vi "Fetch Multi Eval Meas List SEM Margin Area Results.vi"(6 "Area (1)":T2=1, 7 "Offset Frequency (Negative)":i32(ring) items=["Negative", "Positive"], 8 "error in (no error)":errorcluster, 9 "Result Type (Current)":i32(ring) items=["Current"=0, "Average"=1, "Minimum"=5], 10 "Instance (1)":T3=1, 11 "VISA resource name":refnum<visa-resource-name>) -> (0 "error out":errorcluster, 2 "Reliability":i32, 3 "VISA resource name out":refnum<visa-resource-name>)   [LabVIEW 2020, in "Rohde&Schwarz CMXP NR FR2 Measurement.lvlib"]
doc: "Returns spectrum emission mask margin positions for all measured list mode segments.\n\nAttributes:\nRSCMXPNRFR2M_ATTR_FETCH_MULTI_EVAL_MEASUREMENT_LIST_SEM_MARGIN_AREA_NEGATIVE_AVERAGE_RESULTS\nRSCMXPNRFR2M_ATTR_FETCH_MULTI_EVAL_MEASUREMENT_LIST_SEM_MARGIN_AREA_NEGATIVE_CURRENT_RESULTS\nRSCMXPNRFR2M_ATTR_FETCH_MULTI_EVAL_MEASUREMENT_LIST_SEM_MARGIN_AREA_NEGATIVE_MINIMUM_RESULTS\nRSCMXPNRFR2M_ATTR_FETCH_MULTI_EVAL_MEASUREMENT_LIST_SEM_MARGIN_AREA_POSITIVE_AVERAGE_RESULTS\nRSCMXPNRFR2M_ATTR_FETCH_MULTI_EVAL_MEASUREMENT_LIST_SEM_MARGIN_AREA_POSITIVE_CURRENT_RESULTS\nRSCMXPNRFR2M_ATTR_FETCH_MULTI_EVAL_MEASUREMENT_LIST_SEM_MARGIN_AREA_POSITIVE_MINIMUM_RESULTS\n\nRemote-control commands:\nFETCh:NRMMw:MEAS<i>:MEValuation:LIST:SEMask:MARGin:AREA<no>:NEGativ:AVERage?\nFETCh:NRMMw:MEAS<i>:MEValuation:LIST:SEMask:MARGin:AREA<no>:NEGativ:CURRent?\nFETCh:NRMMw:MEAS<i>:MEValuation:LIST:SEMask:MARGin:AREA<no>:NEGativ:MINimum?\nFETCh:NRMMw:MEAS<i>:MEValuation:LIST:SEMask:MARGin:AREA<no>:POSitiv:AVERage?\nFETCh:NRMMw:MEAS<i>:MEValuation:LIST:SEMask:MARGin:AREA<no>:POSitiv:CURRent?\nFETCh:NRMMw:MEAS<i>:MEValuation:LIST:SEMask:MARGin:AREA<no>:POSitiv:MINimum?"
uses:
  <instrlib>/Rohde&Schwarz CMXP NR FR2 Measurement/Rohde&Schwarz CMXP NR FR2 Measurement.lvlib
  <instrlib>/Rohde&Schwarz CMXP NR FR2 Measurement/Private/_Instance.ctl
  <instrlib>/Rohde&Schwarz CMXP NR FR2 Measurement/Private/_Area.ctl
  <instrlib>/Rohde&Schwarz CMXP NR FR2 Measurement/Private/rsidr_core.llb/rsidr_core.lvlib
panel:
  out "SEM Margin Area Results":T1(array[cluster]) {"Margin Pos Y" format="%^.3e"; "Margin Pos X" format="%^.3e"}
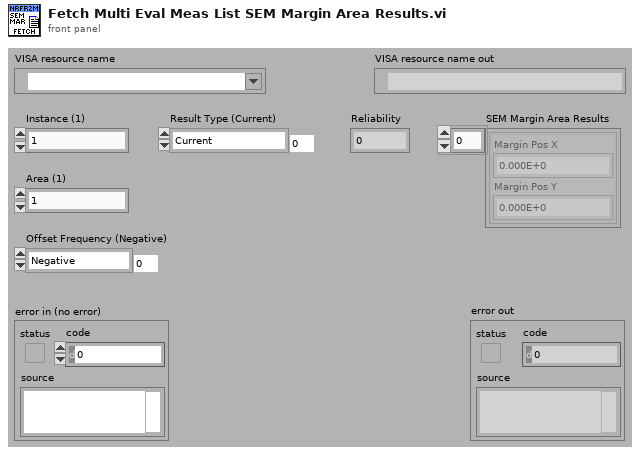
[diagram p1: front panel]
types:
  T1 = cluster{"Margin Pos X":dbl, "Margin Pos Y":dbl}[]
  T2 = typedef "Rohde&Schwarz CMXP NR FR2 Measurement.lvlib/_Area.ctl" = i32
  T3 = typedef "Rohde&Schwarz CMXP NR FR2 Measurement.lvlib/_Instance.ctl" = i32
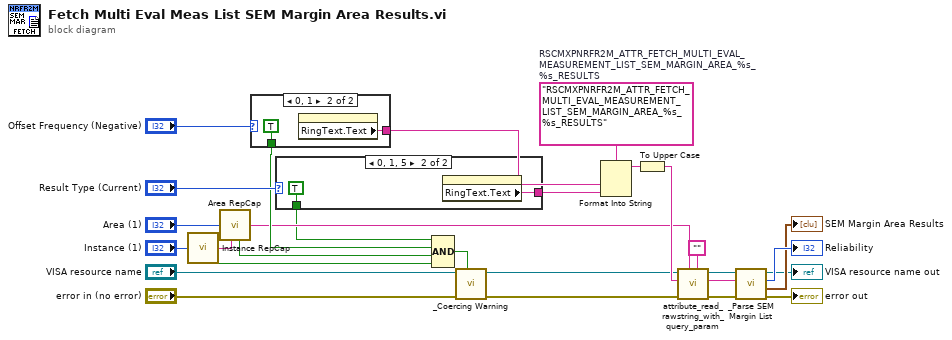
[diagram p0: block diagram]
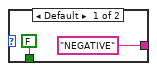
[diagram p2: hidden frame]
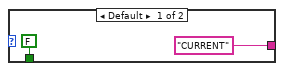
[diagram p3: hidden frame]
diagram:
  w22 = "RSCMXPNRFR2M_ATTR_FETCH_MULTI_EVAL_MEASUREMENT_LIST_SEM_MARGIN_AREA_%s_%s_RESULTS"  # RSCMXPNRFR2M_ATTR_FETCH_MULTI_EVAL_MEASUREMENT_LIST_SEM_MARGIN_AREA_%s_%s_RESULTS
  n1 = call <instrlib>:"Instance RepCap.vi"("Instance In"="Instance (1)") -> ("In Range?"=w24:bool, "RepCap Identifier Out"=w1:string)  [unwired: 1 in]
  n2 = call <instrlib>:"Area RepCap.vi"("SEM Area In"="Area (1)", "RepCap String In (\"\")"=w1) -> ("In Range?"=w23:bool, "RepCap Identifier Out"=w12:string)
  n3 = case shown="0, 1" "Offset Frequency (Negative)" {
    tunnel: ["NEGATIVE" w31] -> w4
    tunnel: [FALSE TRUE] -> w17
    frame Default {
    }
    frame 0, 1 {
      n4 = property on="Offset Frequency (Negative)" class="Ring (strict)"() -> ("RingText.Text"=w31:string)  [unwired: 2 in, 2 out]
    }
  }
  n5 = case shown="0, 1, 5" "Result Type (Current)" {
    tunnel: ["CURRENT" w35] -> w20
    tunnel: [FALSE TRUE] -> w3
    frame Default {
    }
    frame 0, 1, 5 {
      n6 = property on="Result Type (Current)" class="Ring (strict)"() -> ("RingText.Text"=w35:string)  [unwired: 2 in, 2 out]
    }
  }
  n7 = Compound Arithmetic op=AND(w3, w17, w23, w24) -> (w25:bool)
  n8 = call <instrlib>:"_Coercing Warning.vi"("In Range?"=w25, "error in (no error)"="error in (no error)", "VISA resource name"="VISA resource name") -> ("error out"=w15:errorcluster, "VISA resource name out"=w13:refnum<visa-resource-name>)  [unwired: 7 in]
  n9 = Format Into String(format string=w22, w4, w20) -> (resulting string=w19:string)  [unwired: 2 in, 1 out]
  n10 = To Upper Case(1:w19) -> (0:w14:string)
  n11 = call <instrlib>:"attribute_read_rawstring_with_query_param.vi"("Query Parameter (None)"="" ("Empty String Constant"), "Repeated Capability"=w12, "error in"=w15, "Attribute ID"=w14, "VISA resource name"=w13) -> ("error out"=w11:errorcluster, "Raw String out"=w10:string, "VISA resource name out"=w9:refnum<visa-resource-name>)  [unwired: 4 in]
  n12 = call <instrlib>:"_Parse SEM Margin List.vi"("error in (no error)"=w11, "Input String"=w10, "VISA resource name"=w9) -> ("error out"=→"error out":errorcluster, "Results"=→"SEM Margin Area Results":T1, "Reliability"=→"Reliability":i32, "VISA resource name out"=→"VISA resource name out":refnum<visa-resource-name>)  [unwired: 5 in]
